vi "Write Enable Digital Trigger.vi"(8 "error in (no error)":errorcluster, 10 "Enable Digital Trigger":bool, 11 "AnalogInput in":refnum<class "AnalogInput.lvclass">) -> (0 "error out":errorcluster, 3 "AnalogInput out":refnum<class "AnalogInput.lvclass">)   [LabVIEW 2019, in "AnalogInput.lvlib" / "AnalogInput.lvclass"]
uses:
  Library/AnalogInput.lvclass
  Library/AnalogInput.lvclass/AnalogInput.ctl
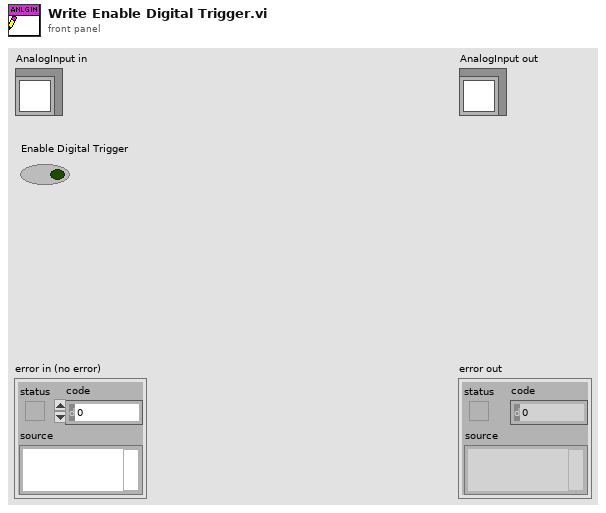
[diagram p1: front panel]
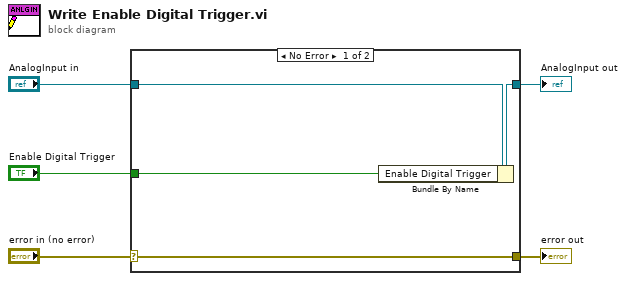
[diagram p0: block diagram]
diagram:
  n1 = case shown="No Error" "error in (no error)" {
    selector: "error in (no error)" -> [w9 w10]
    tunnel: [w9 w10] -> w4
    tunnel: [w7 w11] -> w2
    tunnel: "AnalogInput in" -> [w8 w11]
    tunnel: "Enable Digital Trigger" -> [w6 _]
    frame No Error {
      n2 = Bundle By Name(cluster=w8, "Enable Digital Trigger"=w6) -> (w7:refnum<class "AnalogInput.lvclass">)
    }
    frame Error {
    }
  }
  "error out" <- w4
  "AnalogInput out" <- w2
